vi "Test At Least Two Calls Any Inputs Fail.vi"(8 "error in (no error)":errorcluster, 11 "Test Case In":refnum<class "Expectation Message Test.lvclass">) -> (0 "error out":errorcluster, 3 "Test Case Out":refnum<class "Expectation Message Test.lvclass">)   [LabVIEW 2020, in "Expectation Message Test.lvclass"]
uses:
  Expectation Message Test.lvclass
  C:/Program Files (x86)/National Instruments/LabVIEW 2020/vi.lib/Astemes/LUnit/Test Case.lvclass
  Test Doubles/Test Interface Responsive Mock/Test Interface Mock.lvclass
  C:/git/astemes-lmock/source/Framework/Mock/LMock Mock.lvclass
  source/Expectations/At Least/At Least Ignore Inputs.vi
  Expectation Message Test.lvclass/Expectation Message Test.ctl
  C:/git/astemes-lmock/tests/Test Doubles/Test Interface Responsive Mock/Test Interface Mock.lvclass
  C:/git/astemes-lmock/tests/Test Doubles/Test Interface/Test Interface.lvclass
  Expectation Test/Expectation Test.lvclass
  source/Framework/LMock API.lvlib
  source/Expectations/At Least/At Least.lvlib
  C:/git/astemes-lmock/tests/Expectation Test/Expectation Test.lvclass
  C:/Program Files (x86)/National Instruments/LabVIEW 2020/vi.lib/Astemes/LUnit/LUnit Runnable.lvclass
  C:/git/astemes-lmock/tests/Verify Message Test/Expectation Message Test.lvclass
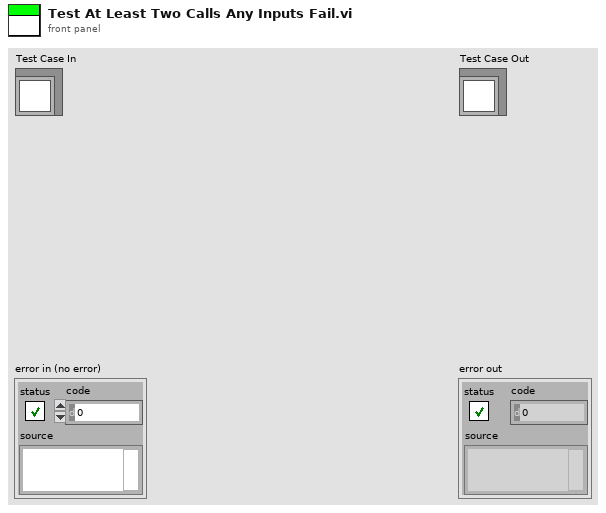
[diagram p1: front panel]
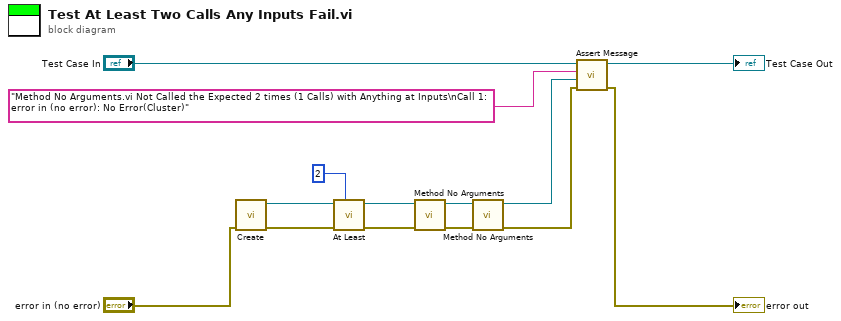
[diagram p0: block diagram]
diagram:
  n1 = call "Create.vi"("error in (no error)"="error in (no error)") -> ("error out"=w11:errorcluster, "Test Interface Mock Out"=w9:refnum<class "Test Interface Mock.lvclass">)  [unwired: 9 in]
  n2 = call-poly "At Least.vi"("Minimum Number of Calls"=u32 2 ("Expected Number of Calls"), "error in (no error)"=w11, "Mock in"=w9) -> ("error out"=w10:errorcluster, "Mock out"=w8:refnum<class "Test Interface Mock.lvclass">)  [unwired: 7 in]
  n3 = call-dynamic "Method No Arguments.vi"("error in (no error)"=w10, "Mock In"=w8) -> ("error out"=w7:errorcluster, "Mock Out"=w4:refnum<class "Test Interface Mock.lvclass">)  [unwired: 8 in]
  n4 = call-dynamic "Method No Arguments.vi"("error in (no error)"=w7, "Mock In"=w4) -> ("error out"=w2:errorcluster, "Mock Out"=w1:refnum<class "Test Interface Mock.lvclass">)  [unwired: 8 in]
  n5 = call "Assert Message.vi"("error in (no error)"=w2, "Mock"=w1, "Message"="Method No Arguments.vi Not Called the Expected 2 times (1 Calls) with Anything at Inputs\nCall 1: error in (no error): No Error(Cluster)", "LUnit Test Case In"="Test Case In") -> ("error out"=→"error out":errorcluster, "LUnit Test Case Out"=→"Test Case Out":refnum<class "Expectation Message Test.lvclass">)  [unwired: 6 in]
